vi "Parse.vi"(8 "Error In":errorcluster, 11 "object in":refnum<class "2022_8.lvclass">) -> (0 "Error Out":errorcluster, 3 "object out":refnum<class "2022_8.lvclass">)   [LabVIEW 2023, in "2022_8.lvclass"]
uses:
  2022_8.lvclass
  2022_8.lvclass/2022_8.ctl
  <vilib>/Utility/error.llb/Trim Whitespace One-Sided.vi
  <userlib>/_OpenG.lib/string/string.llb/openg_string.lvlib
panel:
  out "Map":u8[][](array[numeric])
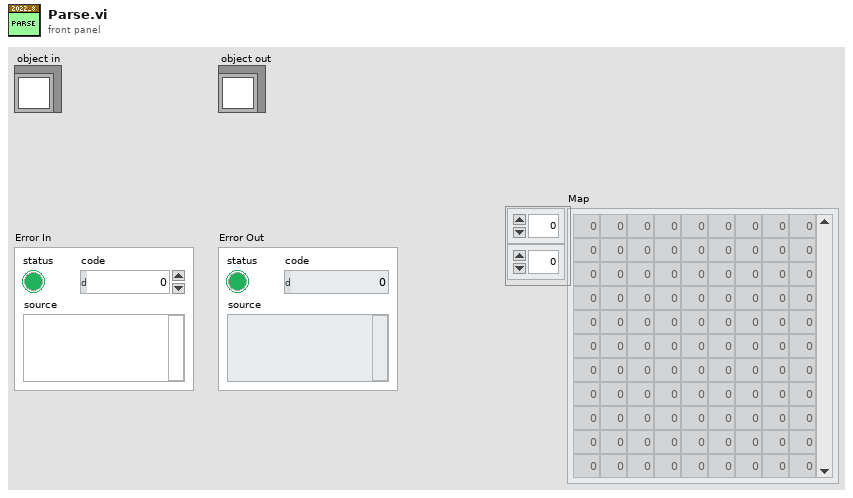
[diagram p1: front panel]
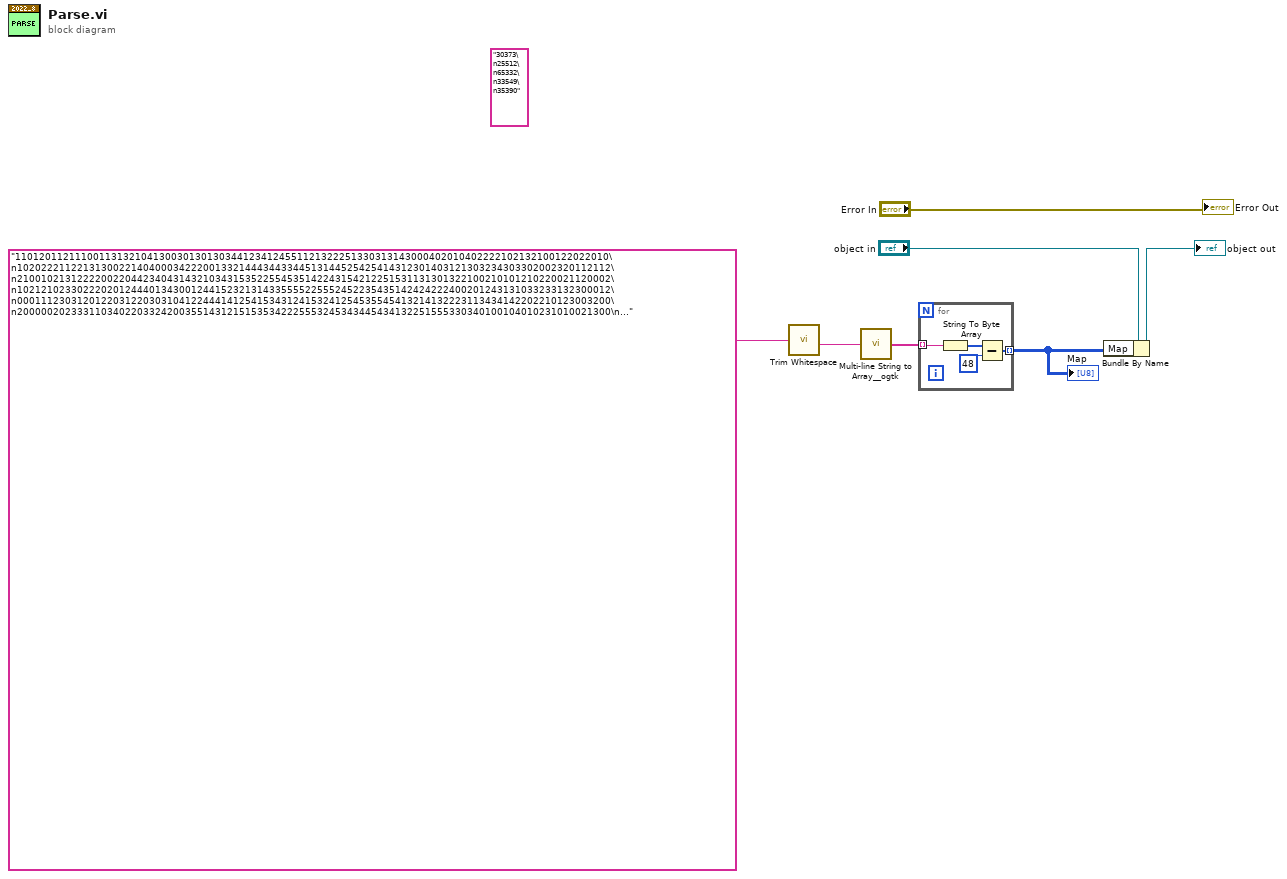
[diagram p0: block diagram]
diagram:
  (unwired) "30373\n25512\n65332\n33549\n35390"
  n1 = call <vilib>:"Trim Whitespace.vi"("string"="110120112111001131321041300301301303441234124551121322251330313143000402010402222102132100122022010\n102022211221313002214040003422200133214443443344513144525425414312301403121303234303302002320112112\n210010213122220022044234043143210343153522554535142243154212251531131301322100210101210220021120002\n102121023302220201244401343001244152321314335555225552452235435142424222400201243131033233132300012\n000111230312012203122030310412244414125415343124153241254535545413214132223113434142202210123003200\n200000202333110340220332420035514312151535342225553245343445434132251555330340100104010231010021300\n...") -> ("trimmed string"=w4:string)  [unwired: 1 in]
  n2 = call <userlib>:"Multi-line String to Array__ogtk.vi"("string"=w4) -> ("lines"=w3:string[])
  n3 = for {
    tunnel: w3 -> [w11] mode=indexing
    tunnel: [w8] -> w2 mode=indexing
    n4 = String To Byte Array(string=w11) -> (unsigned byte array=w10:u8[])
    n5 = Subtract(x=w10, y=u8 48) -> (x-y=w8:u8[])
  }
  "Map" <- w2
  n6 = Bundle By Name(cluster="object in", "Map"=w2) -> (→"object out":refnum<class "2022_8.lvclass">)
  "Error Out" <- "Error In"
